vi "extract_data.vi"(11 "Data IN":u16[](array[numeric])) -> (2 "Error":bool, 3 "Read Data":T1 {"Conductivity [uS/cm]" format="%#_f"; "Pressure [bar]" format="%#_f"; "PH" format="%#_f"; "Water Level [L]" format="%#_f"; "Temperature [°C]" format="%#_f"})   [LabVIEW 2025, in "TanksPlcDriver.lvlib"]
uses:
  TanksPlcDriver.lvlib
  TypeDefs/ReadData.ctl
panel:
  # "note: Connected/Disconnected status is determined from data \nreceived. If the whole read data block is read as 0 the sensor is flagged\nas not connected! IO-Link has special registers for identifying sensor\nconnection status but these are in separate data ranges and all data 0\nshould be reliable as the system will not operate with water\ntemperatures of 0°C"
  # "Global constants"
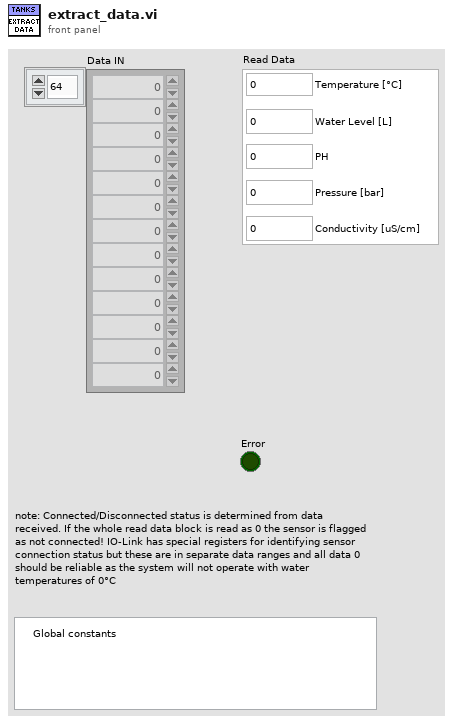
[diagram p1: front panel]
types:
  T1 = typedef "TanksPlcDriver.lvlib/ReadData.ctl" = cluster{"Temperature [°C]":dbl, "Water Level [L]":dbl, "PH":dbl, "Conductivity [uS/cm]":dbl, "Pressure [bar]":dbl}
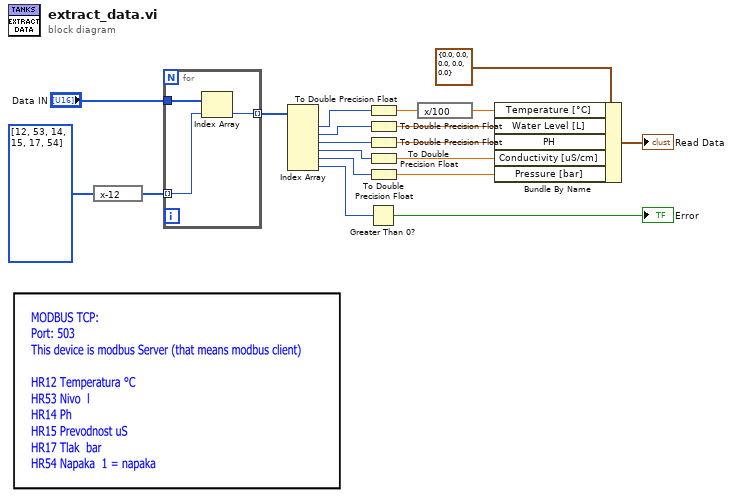
[diagram p0: block diagram]
diagram:
  n1 = expression code="x-12"(u16[] [12, 53, 14, 15, 17, 54] ("starting address")) -> (w15:u16[])
  n2 = for {
    tunnel: "Data IN" -> [w22]
    tunnel: w15 -> [w21] mode=indexing
    tunnel: [w20] -> w9 mode=indexing
    n3 = Index Array(array=w22, index=w21) -> (element=w20:u16)
  }
  n4 = Index Array(array=w9) -> (element #1=w14:u16, element #2=w13:u16, element #3=w12:u16, element #4=w11:u16, element #5=w10:u16, element #6=w8:u16)  [unwired: 6 in]
  n5 = Greater Than 0?(x=w8) -> (x > 0?=→"Error":bool)
  n6 = To Double Precision Float(number=w14) -> (double precision float=w6:dbl)
  n7 = To Double Precision Float(number=w13) -> (double precision float=w5:dbl)
  n8 = To Double Precision Float(number=w12) -> (double precision float=w4:dbl)
  n9 = To Double Precision Float(number=w11) -> (double precision float=w3:dbl)
  n10 = To Double Precision Float(number=w10) -> (double precision float=w2:dbl)
  n11 = expression code="x/100"(w6) -> (w1:dbl)
  n12 = Bundle By Name(cluster=T1 {"Temperature [°C]"=0.0, "Water Level [L]"=0.0, "PH"=0.0, "Conductivity [uS/cm]"=0.0, "Pressure [bar]"=0.0} ("Read Data"), "Temperature [°C]"=w1, "Water Level [L]"=w5, "PH"=w4, "Conductivity [uS/cm]"=w3, "Pressure [bar]"=w2) -> (→"Read Data":T1)
